vi "DCC_AskUserForModules.vi"(6 "Array Of\nUsable Moduls":T1[](array[typedef]), 7 "Serial Number In":string[](array[string])=["150 N", "150 N"], 8 "error in":errorcluster={"status"=FALSE, "code"=0, "source"="no error"}, 10 "Array of Modules":i16[](array[numeric]), 11 "DLL Path":path=path "C:/Program Files (x86)/BH/SPCM/DLL/spcm64.dll") -> (0 "error out":errorcluster, 1 "Serial Number":string[](array[string])=["", "150 N"], 3 "DLL Path":path=path "C:/Program Files (x86)/BH/SPCM/DLL/spcm64.dll", 4 "Name of Modules":string[](array[string]), 5 "Active Module No":i16[](array[numeric]))   [LabVIEW 2019]
doc: "This function scans the system after usable modules. These modules will then be listed and the user can choose which one will be used in the running application.\nThe return value is an array which contains the module number of the choosen modules.\nThis function is not intend to use in parallel.\n\nMay 2019\nFrank Quadt\ninfo@becker-hickl.com"
uses:
  DCC_Controls/DCC_ModuleInfoCluster.ctl
panel:
  in  "OK":bool
  out "Module Type(s)":string[](array[string])=["", "150 N"]
  in  "Modules":T2
  in  "Name of Modules":string[](array[string])=["Detector 1", "Detector 2", "Detector 3", "Detector 4 ", "Detector 5", "Detector 6", "Detector 7", "Detector 8"]
  # "Please Choose the Becker & Hickl DCC Module to use"
  # "(c) 2021 Becker & Hickl GmbH\n     ALL RIGHTS RESERVED."
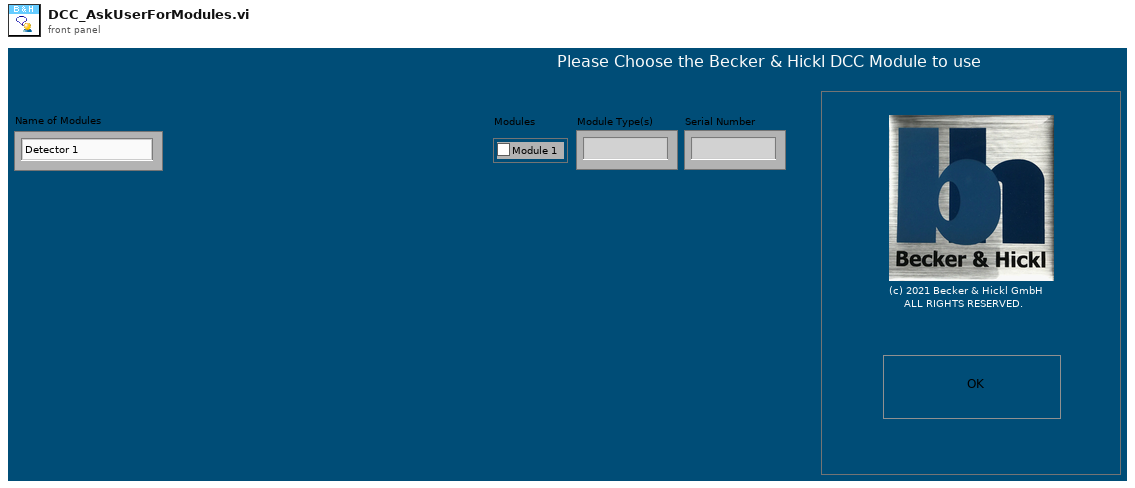
[diagram p1: front panel]
types:
  T1 = typedef "DCC_ModuleInfoCluster.ctl" = cluster{"Module Type":i16, "Bus Number":i16, "Slot Number":i16, "In Use?":i16, "Init":i16, "Base I/O Address":u16, "Module Serial Number":string}
  T2 = cluster{"Module 1":bool, "Module 2":bool, "Module 3":bool, "Module 4":bool, "Module 5":bool, "Module 6":bool, "Module 7":bool, "Module 8":bool}
  T3 = enum32{"Invalid", "Standard", "Closed", "Hidden", "Minimized", "Maximized"}
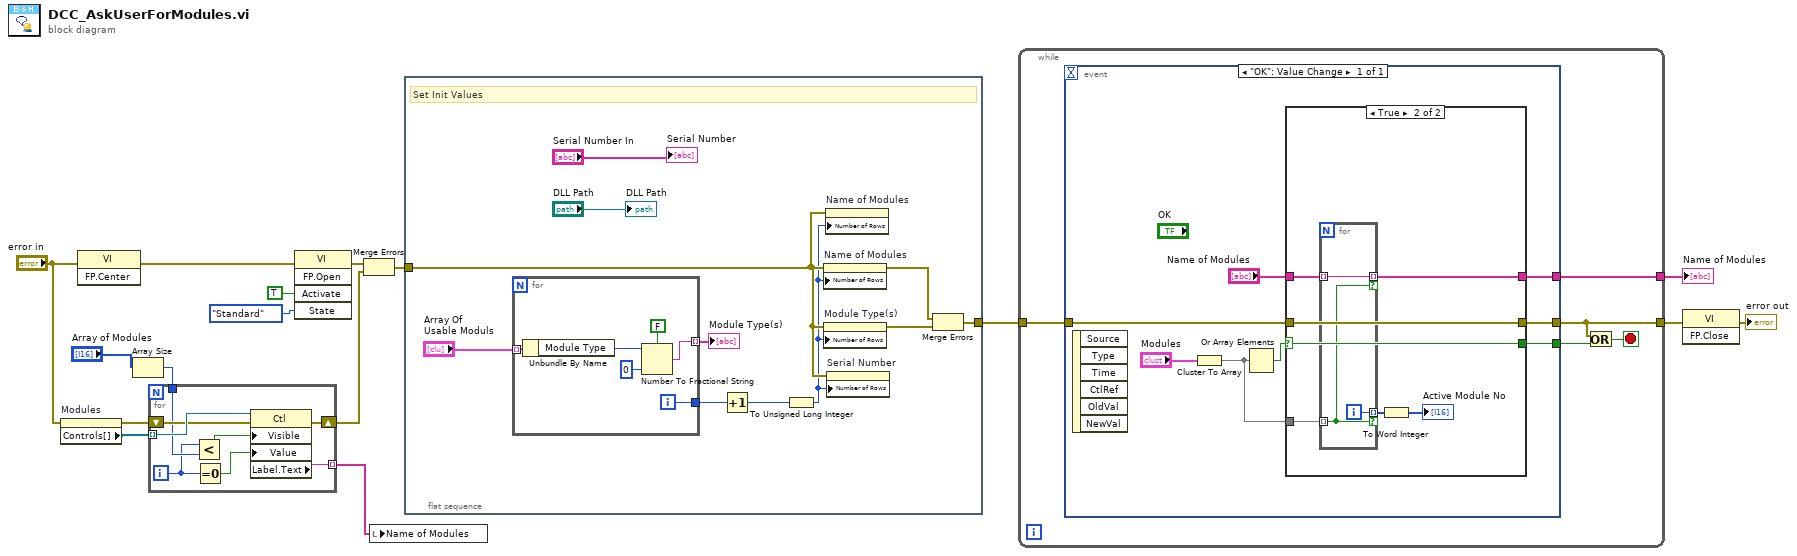
[diagram p0: block diagram]
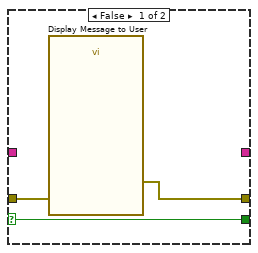
[diagram p2: hidden frame]
diagram:
  n1 = property on="Modules" class="Clust (strict)"(error in="error in") -> (error out=w10:errorcluster, "Controls[]"=w9:refnum<vi>[])  [unwired: 1 in, 1 out]
  n2 = invoke class="VI" method="FP.Center"(error in="error in") -> (error out=w15:errorcluster)  [unwired: 2 in, 2 out]
  n3 = Array Size(array="Array of Modules") -> (size(s)=w5:i32)
  n4 = for {
    tunnel: w9 -> [w24] mode=indexing
    shift-right: [w23] -> w3
    shift-left: w10 -> [w22]
    tunnel: w5 -> [w21]
    tunnel: [w18] -> w1 mode=indexing
    i -> [w20]
    n5 = Less?(x=w20, y=w21) -> (x < y?=w17:bool)
    n6 = Equal To 0?(x=w20) -> (x = 0?=w19:bool)
    n7 = property class="Ctl"(reference=w24, error in=w22, "Visible"=w17, "Value"=w19) -> (error out=w23:errorcluster, "Label.Text"=w18:string)  [unwired: 1 out]
  }
  n8 = invoke class="VI" method="FP.Open"(error in=w15, "Activate"=TRUE ("Activate?"), "State"=T3."Standard") -> (error out=w12:errorcluster)  [unwired: 2 in, 4 out]
  n9 = Merge Errors(w12, w3) -> (w11:errorcluster)
  n10 = local write "Name of Modules"(w1) -> ()
  n11 = flat-sequence {
    tunnel: [w31] -> w7
    tunnel: w11 -> [w26]
    frame #0 {
      # "Set Init Values"
      n12 = for {
        tunnel: "Array Of\nUsable Moduls" -> [w41] mode=indexing
        tunnel: [w39] -> w34 mode=indexing
        tunnel: [w40] -> w33
        i -> [w40]
        n13 = Unbundle By Name(w41) -> ("Module Type"=w38:i16)
        n14 = Number To Fractional String(use system decimal point (T)=FALSE, number=w38, precision (6)=i16 0) -> (F-format string=w39:string)  [unwired: 1 in]
      }
      "Module Type(s)" <- w34
      n15 = Increment(x=w33) -> (x+1=w27:i32)
      n16 = To Unsigned Long Integer(number=w27) -> (unsigned 32bit integer=w25:u32)
      n17 = property on="Name of Modules" class="Arr (strict)"(error in=w26, "Number of Rows"=w25) -> (error out=w32:errorcluster)  [unwired: 1 in, 1 out]
      n18 = property on="Module Type(s)" class="Arr (strict)"(error in=w26, "Number of Rows"=w25) -> (error out=w30:errorcluster)  [unwired: 1 in, 1 out]
      n19 = property on="Name of Modules" class="Arr (strict)"(error in=w26, "Number of Rows"=w25) -> ()  [unwired: 1 in, 2 out]
      n20 = property on="Serial Number" class="Arr (strict)"(error in=w26, "Number of Rows"=w25) -> ()  [unwired: 1 in, 2 out]
      n21 = Merge Errors(w32, w30) -> (w31:errorcluster)
      "DLL Path" <- "DLL Path"
      "Serial Number" <- "Serial Number In"
    }
  }
  n22 = while {
    tunnel: w7 -> [w45]
    tunnel: [w44] -> w6
    tunnel: [w42] -> w2
    stop <- w46 stop-if-true
    n23 = event shown="[0] \"OK\": Value Change" {
      selector: _ -> [_]
      dyn-events: _ -> [_]
      timeout: _ -> [_]
      tunnel: [w47] -> w42
      tunnel: w45 -> [w53]
      tunnel: [w52] -> w44
      tunnel: [w51] -> w43
      event "OK": Value Change {
        n24 = event-data() -> ()  [unwired: 1 in, 6 out]
        n25 = Cluster To Array(cluster="Modules") -> (array=w49:bool[])
        n26 = Or Array Elements(Boolean array=w49) -> (logical OR=w54:bool)
        n27 = case shown="True" w54 {
          selector: w54 -> [w55 w63]
          tunnel: w53 -> [w57 w64]
          tunnel: [w56 w64] -> w52
          tunnel: [w55 w63] -> w51
          tunnel: w49 -> [_ w60]
          tunnel: "Name of Modules" -> [_ w59]
          tunnel: [_ w58] -> w47
          frame False {
            n28 = call "Display Message to User"("error in (no error)"=w57) -> ("error out"=w56:errorcluster)  [unwired: 9 in, 1 out]
          }
          frame True {
            n29 = for {
              tunnel: [w67] -> w62 mode=indexing if=w65
              tunnel: w60 -> [w65] mode=indexing
              tunnel: w59 -> [w66] mode=indexing
              tunnel: [w66] -> w58 mode=indexing if=w65
              i -> [w67]
            }
            n30 = To Word Integer(number=w62) -> (16bit integer=→"Active Module No":i16[])
          }
        }
      }
    }
    n31 = Or(x=w44, y=w43) -> (x .or. y?=w46:bool)
  }
  "Name of Modules" <- w2
  n32 = invoke class="VI" method="FP.Close"(error in=w6) -> (error out=→"error out":errorcluster)  [unwired: 2 in, 2 out]
